vi "AddHandler.vi"(0 "Config in":T1, 5 "Server Index":i32, 7 "HandlerName":string, 9 "Extensions":string[](array[string]), 11 "error in (no error)":errorcluster) -> (4 "Config out":T1, 15 "error out":errorcluster)   [LabVIEW 2017]
uses:
  <vilib>/WebServerConfig/Config.ctl
  <vilib>/WebServerConfig/Server.ctl
  <vilib>/WebServerConfig/Alias.ctl
  <vilib>/WebServerConfig/ErrorDocument.ctl
  <vilib>/WebServerConfig/Action.ctl
  <vilib>/WebServerConfig/Redirect.ctl
  <vilib>/WebServerConfig/Interface.ctl
  <vilib>/WebServerConfig/AddHandler.ctl
  <vilib>/WebServerConfig/SSL.ctl
  <vilib>/WebServerConfig/CustomLog.ctl
  <vilib>/WebServerConfig/LoadModule.ctl
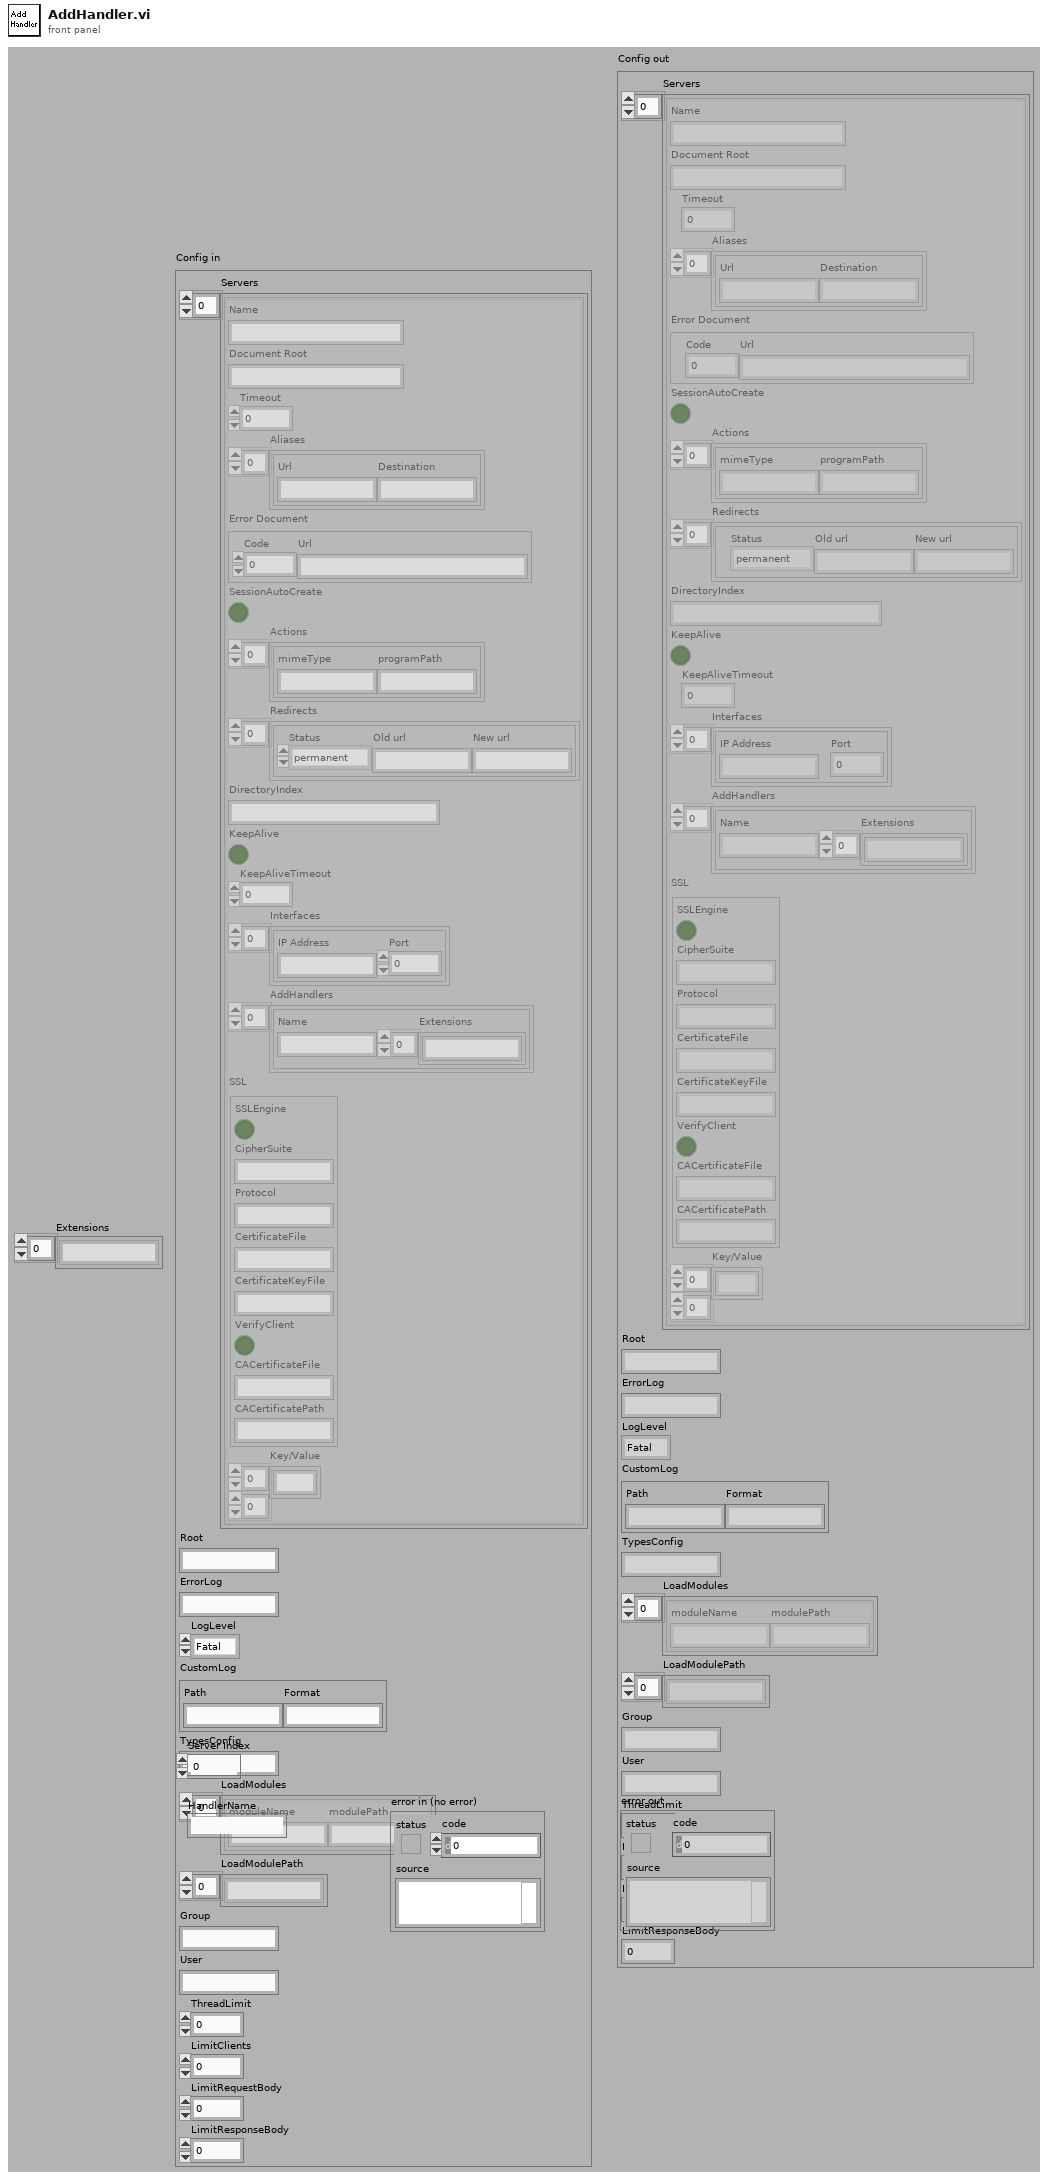
[diagram p1: front panel]
types:
  T1 = typedef "Config.ctl" = cluster{"Servers":T2[], "Root":string, "ErrorLog":string, "LogLevel":enum16{"Fatal", "Error", "Warn", "Info", "Debug", "5", "6", "7", "8", "Verbose"}, "CustomLog":T10, "TypesConfig":string, "LoadModules":T11[], "LoadModulePath":string[], "Group":string, "User":string, "ThreadLimit":u32, "LimitClients":u32, "LimitRequestBody":u32, "LimitResponseBody":u32}
  T2 = typedef "Server.ctl" = cluster{"Name":string, "Document Root":string, "Timeout":u32, "Aliases":T3[], "Error Document":T4, "SessionAutoCreate":bool, "Actions":T5[], "Redirects":T6[], "DirectoryIndex":string, "KeepAlive":bool, "KeepAliveTimeout":u32, "Interfaces":T7[], "AddHandlers":T8[], "SSL":T9, "Key/Value":string[][]}
  T3 = typedef "Alias.ctl" = cluster{"Url":string, "Destination":string}
  T4 = typedef "ErrorDocument.ctl" = cluster{"Code":u16, "Url":string}
  T5 = typedef "Action.ctl" = cluster{"mimeType":string, "programPath":string}
  T6 = typedef "Redirect.ctl" = cluster{"Status":enum16{"permanent", "temp", "seeother", "gone"}, "Old url":string, "New url":string}
  T7 = typedef "Interface.ctl" = cluster{"IP Address":string, "Port":u16}
  T8 = typedef "AddHandler.ctl" = cluster{"Name":string, "Extensions":string[]}
  T9 = typedef "SSL.ctl" = cluster{"SSLEngine":bool, "CipherSuite":string, "Protocol":string, "CertificateFile":string, "CertificateKeyFile":string, "VerifyClient":bool, "CACertificateFile":string, "CACertificatePath":string}
  T10 = typedef "CustomLog.ctl" = cluster{"Path":string, "Format":string}
  T11 = typedef "LoadModule.ctl" = cluster{"moduleName":string, "modulePath":string}
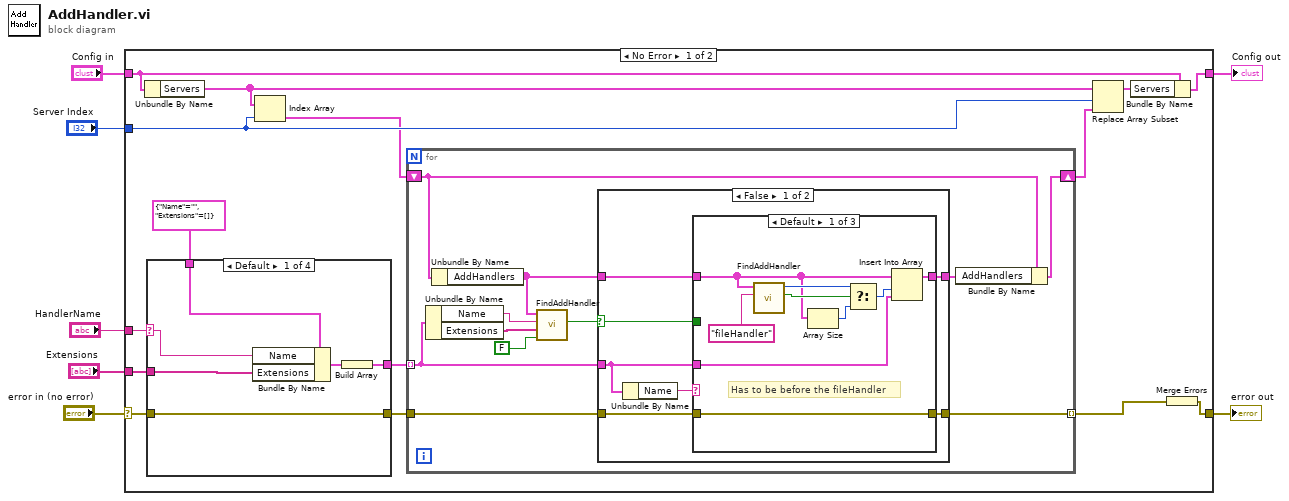
[diagram p0: block diagram]
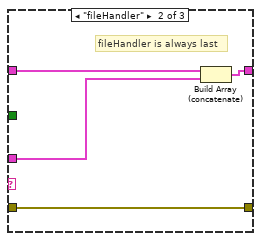
[diagram p2: hidden frame]
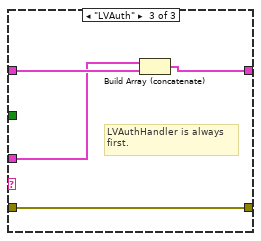
[diagram p3: hidden frame]
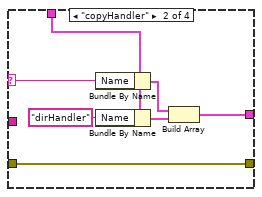
[diagram p5: hidden frame]
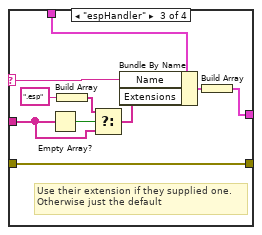
[diagram p6: hidden frame]
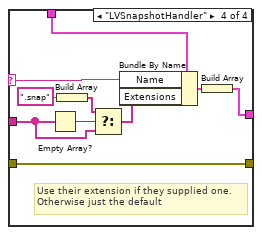
[diagram p7: hidden frame]
diagram:
  n1 = case shown="No Error" "error in (no error)" {
    selector: "error in (no error)" -> [w16 w94]
    tunnel: [w20 w93] -> w6
    tunnel: "Config in" -> [w21 w93]
    tunnel: [w13 w94] -> w4
    tunnel: "HandlerName" -> [w22 _]
    tunnel: "Server Index" -> [w17 _]
    tunnel: "Extensions" -> [w9 _]
    frame No Error {
      n2 = Unbundle By Name(w21) -> ("Servers"=w18:T2[])
      n3 = case shown="Default" w22 {
        selector: w22 -> [w60 w70 w80 w90]
        tunnel: w16 -> [w62 w72 w82 w92]
        tunnel: [w65 w67 w78 w88] -> w12
        tunnel: T8 {"Name"="", "Extensions"=[]} ("AddHandler") -> [w64 w71 w81 w91]
        tunnel: [w62 w72 w82 w92] -> w14
        tunnel: w9 -> [w61 _ w75 w85]
        frame Default {
          n4 = Bundle By Name(cluster=w64, "Name"=w60, "Extensions"=w61) -> (w63:T8)
          n5 = Build Array(w63) -> (w65:T8[])
        }
        frame "copyHandler" {
          n6 = Bundle By Name(cluster=w71, "Name"=w70) -> (w69:T8)
          n7 = Bundle By Name(cluster=w71, "Name"="dirHandler") -> (w68:T8)
          n8 = Build Array(w69, w68) -> (w67:T8[])
        }
        frame "espHandler" {
          # "Use their extension if they supplied one.\nOtherwise just the default"
          n9 = Empty Array?(array=w75) -> (empty?=w76:bool)
          n10 = Build Array(".esp") -> (w74:string[])
          n11 = Select(t=w74, s=w76, f=w75) -> (s? t:f=w73:string[])
          n12 = Bundle By Name(cluster=w81, "Name"=w80, "Extensions"=w73) -> (w79:T8)
          n13 = Build Array(w79) -> (w78:T8[])
        }
        frame "LVSnapshotHandler" {
          # "Use their extension if they supplied one.\nOtherwise just the default"
          n14 = Empty Array?(array=w85) -> (empty?=w86:bool)
          n15 = Build Array(".snap") -> (w84:string[])
          n16 = Select(t=w84, s=w86, f=w85) -> (s? t:f=w83:string[])
          n17 = Bundle By Name(cluster=w91, "Name"=w90, "Extensions"=w83) -> (w89:T8)
          n18 = Build Array(w89) -> (w88:T8[])
        }
      }
      n19 = Index Array(array=w18, index=w17) -> (element=w11:T2)
      n20 = for {
        tunnel: w14 -> [w30]
        tunnel: w12 -> [w27] mode=indexing
        shift-right: [w32] -> w10
        shift-left: w11 -> [w33]
        tunnel: [w29] -> w8 mode=indexing
        n21 = Unbundle By Name(w27) -> ("Name"=w26:string, "Extensions"=w25:string[])
        n22 = Unbundle By Name(w33) -> ("AddHandlers"=w28:T8[])
        n23 = call <vilib>:"FindAddHandler.vi"("ByNameOnly?"=FALSE, "Extensions"=w25, "Name"=w26, "AddHandlers"=w28) -> ("Found"=w24:bool)  [unwired: 6 in, 1 out]
        n24 = case shown="False" w24 {
          selector: w24 -> [w36 _]
          tunnel: w28 -> [w40 w59]
          tunnel: w27 -> [w35 _]
          tunnel: [w39 w59] -> w31
          tunnel: [w37 w58] -> w29
          tunnel: w30 -> [w38 w58]
          frame False {
            n25 = Unbundle By Name(w35) -> ("Name"=w34:string)
            n26 = case shown="Default" w34 {
              tunnel: w40 -> [w42 w53 w57]
              tunnel: [w48 w52 w56] -> w39
              tunnel: w35 -> [w47 w51 w55]
              tunnel: w38 -> [w49 w50 w54]
              tunnel: [w49 w50 w54] -> w37
              tunnel: w36 -> [_ _ _]
              frame Default {
                # "Has to be before the fileHandler"
                n27 = call <vilib>:"FindAddHandler.vi"("Name"="fileHandler", "AddHandlers"=w42) -> ("Found"=w45:bool, "Index"=w44:i32)  [unwired: 8 in]
                n28 = Array Size(array=w42) -> (size(s)=w41:i32)
                n29 = Select(t=w44, s=w45, f=w41) -> (s? t:f=w46:i32)
                n30 = Insert Into Array(array=w42, index=w46, new element=w47) -> (w48:T8[])
              }
              frame "fileHandler" {
                # "fileHandler is always last"
                n31 = Build Array (concatenate)(w53, w51) -> (w52:T8[])
              }
              frame "LVAuth" {
                # "LVAuthHandler is always\nfirst."
                n32 = Build Array (concatenate)(w55, w57) -> (w56:T8[])
              }
            }
          }
          frame True {
          }
        }
        n33 = Bundle By Name(cluster=w33, "AddHandlers"=w31) -> (w32:T2)
      }
      n34 = Replace Array Subset(array=w18, new element=w10, index=w17) -> (w19:T2[])
      n35 = Bundle By Name(cluster=w21, "Servers"=w19) -> (w20:T1)
      n36 = Merge Errors(w8) -> (w13:errorcluster)
    }
    frame Error {
    }
  }
  "Config out" <- w6
  "error out" <- w4
